vi "Periodic Tasks.vi"(8 "error in":errorcluster) -> ()   [LabVIEW 2015]
doc: "This VI runs in parallel to other tasks. It can contain as many user-defined periodic loops as you need. These can carry out PID or other sorts of timed response."
uses:
  Sprocket/lib/Sprocket.lvlib
panel:
  out "error out":errorcluster
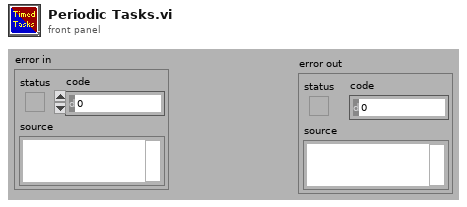
[diagram p1: front panel]
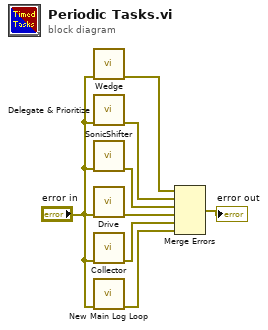
[diagram p0: block diagram]
diagram:
  n1 = call "Wedge.vi"("error in"="error in") -> ("error out"=w2:errorcluster)  [unwired: 10 in]
  n2 = call "Delegate & Prioritize.vi"("error in (no error)"="error in") -> ("error out"=w4:errorcluster)  [unwired: 10 in]
  n3 = call "SonicShifter.vi"("error in"="error in") -> ("error out"=w5:errorcluster)  [unwired: 10 in]
  n4 = call "Drive.vi"("error in"="error in") -> ("error out"=w7:errorcluster)  [unwired: 10 in]
  n5 = call "Collector.vi"("error in"="error in") -> ("error out"=w6:errorcluster)  [unwired: 10 in]
  n6 = call "New Main Log Loop.vi"("error in (no error)"="error in") -> ("error out"=w3:errorcluster)  [unwired: 10 in]
  n7 = Merge Errors(w2, w4, w5, w7, w6, w3) -> (→"error out":errorcluster)
